vi "ServiceStatusSignals.Compile.vi"(8 "error in (no error)":errorcluster, 10 "Settings":T1[](array[typedef]) {"Signal.Cmd.Refs"."Signal Refs" format="%.0x"; "Signal.Cmd.Info"."Signals"."Byte Order" items=["Little Endian", "Big Endian"]; "Signal.Cmd.Info"."Signals"."Data Type" items=["Signed", "Unsigned", "IEEE Float"]; "Settings.Refs"."Signal Refs" format="%.0x"; "Signal.Resp.Refs"."Signal Refs" format="%.0x"; "Signal.Resp.Info"."Signals"."Byte Order" items=["Little Endian", "Big Endian"]; "Signal.Resp.Info"."Signals"."Data Type" items=["Signed", "Unsigned", "IEEE Float"]; "Trigger.Refs"."Signal Refs" format="%.0x"; "Status.Refs"."Signal Refs" format="%.0x"}) -> (0 "error out":errorcluster, 2 "Refs":T7 {"VS Refs" format="%.0x"}, 3 "Status Lookup":variant)   [LabVIEW 2019, in "Diagnostics Addon System Explorer.lvlib"]
uses:
  Diagnostics Addon System Explorer.lvlib
  <vilib>/NI VeriStand/Custom Device API/Custom Device Item Ref.ctl
  Types/Service.Export.ctl
  Types/Frame.Ref.ctl
  Addon Shared/Types/Type.ctl
  Addon Shared/Types/Frame.Compile.ctl
  Addon Shared/Types/Signal.ctl
  Addon Shared/Types/ServiceChannels.LookupType.ctl
  Addon Shared/SubVIs/Constants.vi
  <vilib>/NI VeriStand/Custom Device API/Custom Device API.lvlib
  Addon Shared/Diagnostics Addon Shared.lvlib
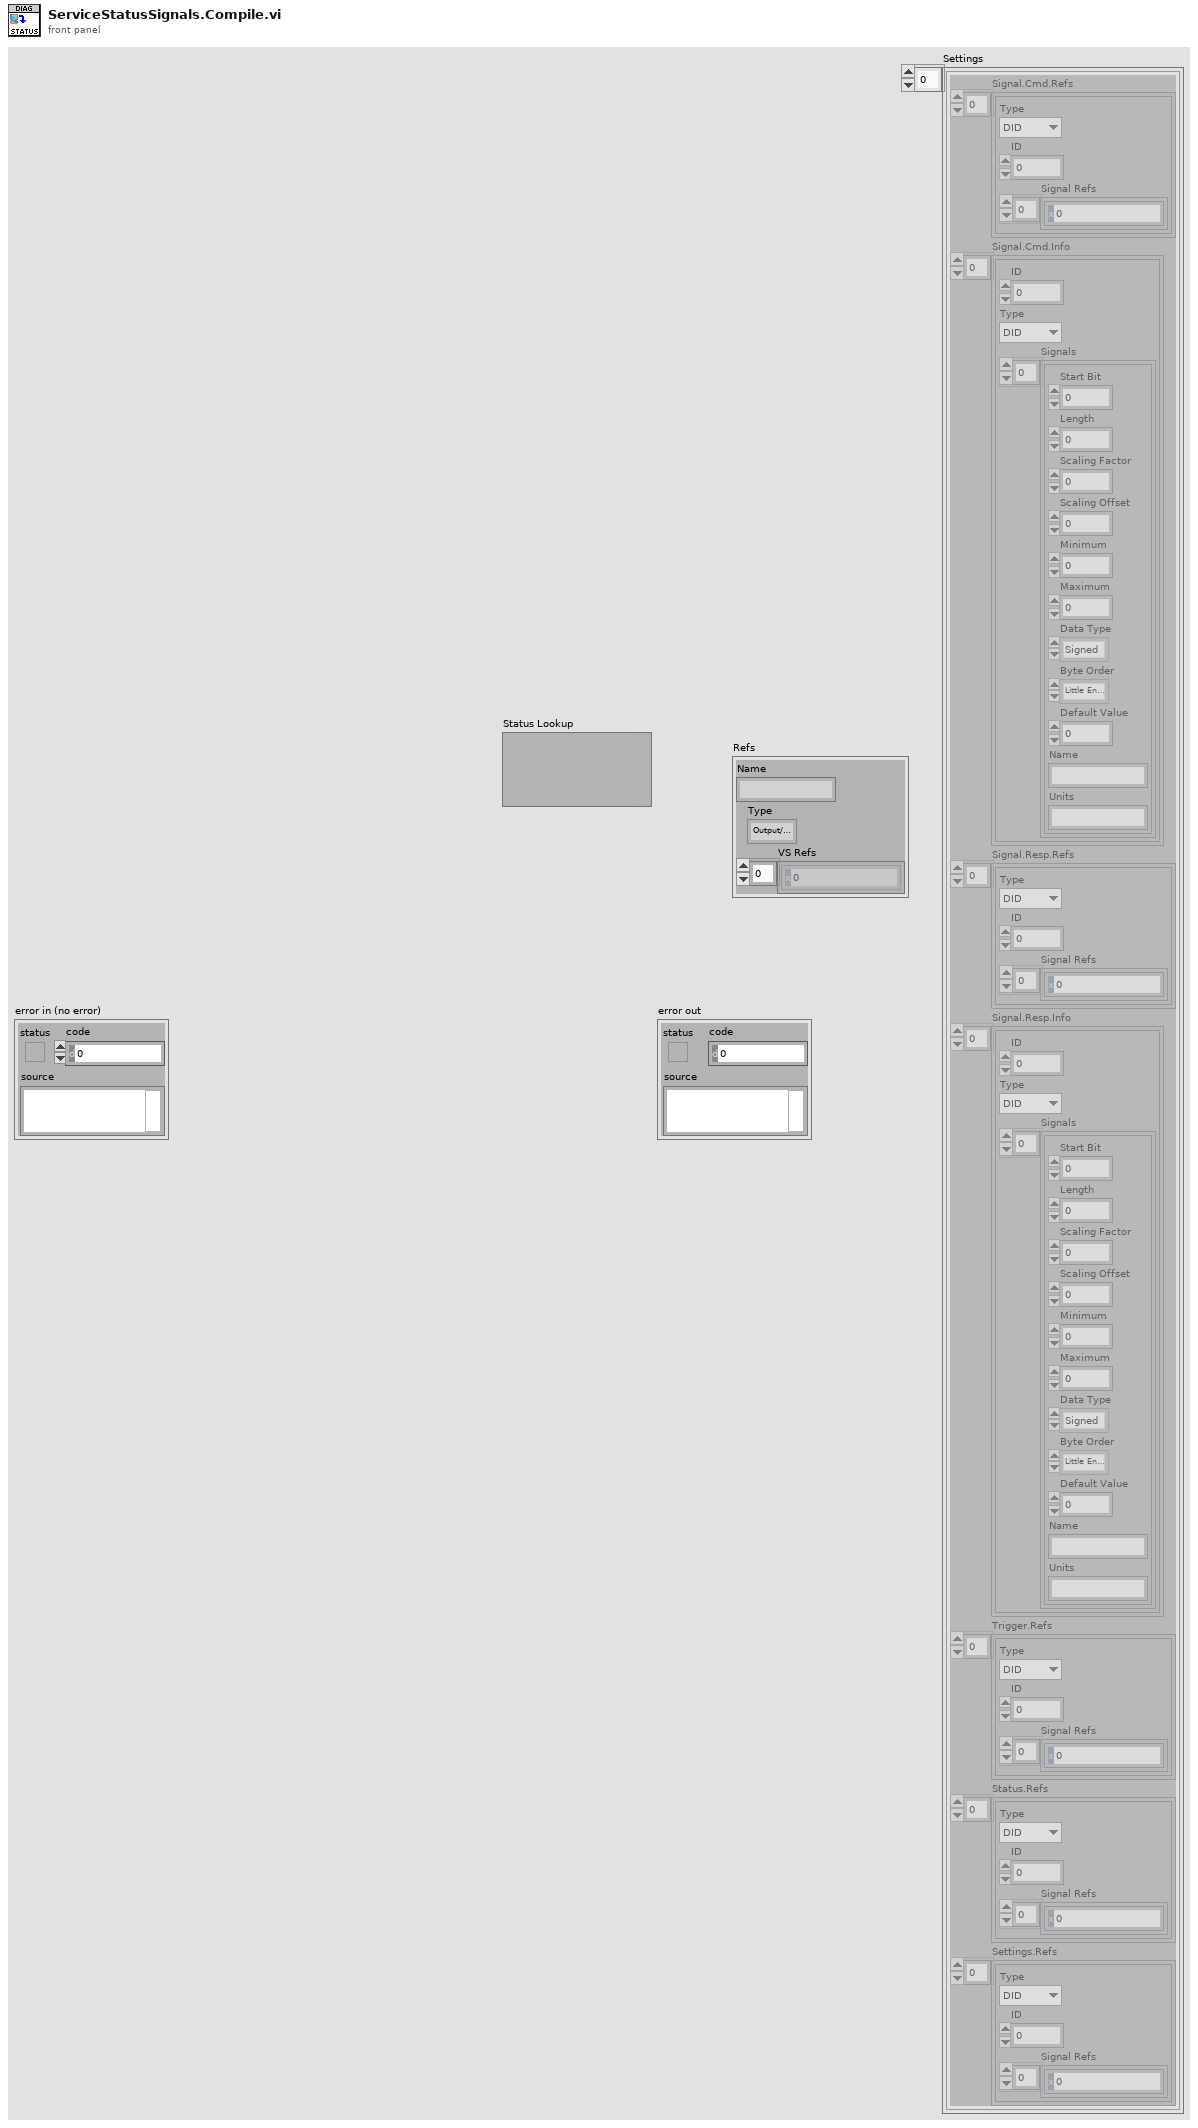
[diagram p1: front panel]
types:
  T1 = typedef "Diagnostics Addon System Explorer.lvlib/Service.Export.ctl" = cluster{"Signal.Cmd.Refs":T2[], "Signal.Cmd.Info":T5[], "Signal.Resp.Refs":T2[], "Signal.Resp.Info":T5[], "Trigger.Refs":T2[], "Status.Refs":T2[], "Settings.Refs":T2[]}
  T2 = typedef "Diagnostics Addon System Explorer.lvlib/Frame.Ref.ctl" = cluster{"Type":T3, "ID":u32, "Signal Refs":T4[]}
  T3 = typedef "Diagnostics Addon Shared.lvlib/Type.ctl" = enum16{"DID", "CDID", "PID", "CPID", "Read Memory", "Write Memory", "IO Control", "Routine Start", "Routine Request", "Routine Stop", "User Defined", "DTC Control", "Clear DTCs", "Read DTCs", "Start DTCs", "DTC Change Count", "Tester Present", "Unlock ECU", "Reset ECU", "Diag Session Control", "Communication Control", "DPID Control", "Poll Control", "Diag CAN Control"}
  T4 = typedef "Custom Device API.lvlib/Custom Device Item Ref.ctl" = u64
  T5 = typedef "Diagnostics Addon Shared.lvlib/Frame.Compile.ctl" = cluster{"ID":u32, "Type":T3, "Signals":T6[]}
  T6 = typedef "Diagnostics Addon Shared.lvlib/Signal.ctl" = cluster{"Start Bit":u32, "Length":u32, "Scaling Factor":dbl, "Scaling Offset":dbl, "Minimum":dbl, "Maximum":dbl, "Data Type":u32, "Byte Order":u32, "Default Value":dbl, "Name":string, "Units":string}
  T7 = cluster{"Name":string, "Type":enum16{"Output/Write", "Input/Read", "Input/ReadWrite"}, "VS Refs":T4[]}
  T8 = enum16{"Output/Write", "Input/Read", "Input/ReadWrite"}
  T9 = typedef "Diagnostics Addon Shared.lvlib/ServiceChannels.LookupType.ctl" = cluster{"Offset":i32}
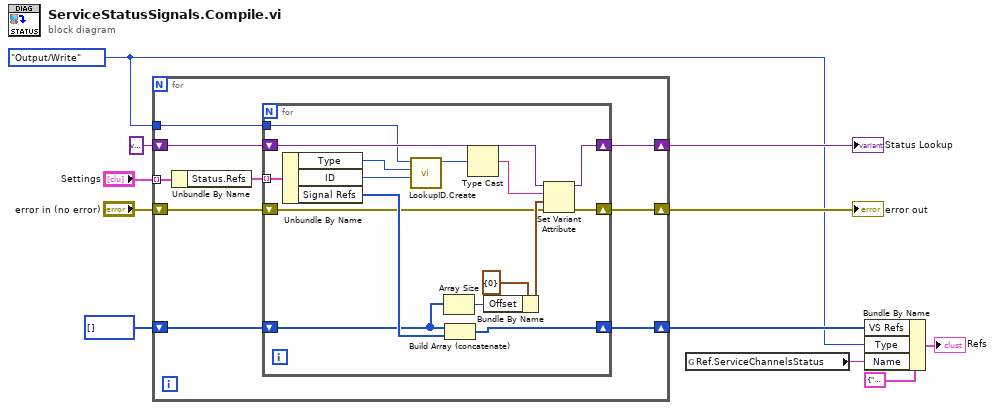
[diagram p0: block diagram]
diagram:
  w1 = T8."Output/Write" ("Type")
  n1 = for {
    shift-right: [w15] -> w4
    shift-left: "error in (no error)" -> [w20]
    shift-right: [w19] -> w10
    shift-left: variant ("Lookup In") -> [w17]
    shift-right: [w16] -> w5
    shift-left: T4[] [] -> [w18]
    tunnel: "Settings" -> [w14] mode=indexing
    tunnel: w1 -> [w12]
    n2 = Unbundle By Name(w14) -> ("Status.Refs"=w13:T2[])
    n3 = for {
      tunnel: w13 -> [w30] mode=indexing
      shift-right: [w31] -> w19
      shift-left: w17 -> [w35]
      shift-right: [w33] -> w15
      shift-left: w20 -> [w26]
      shift-right: [w29] -> w16
      shift-left: w18 -> [w27]
      tunnel: w12 -> [w23]
      n4 = Unbundle By Name(w30) -> ("Type"=w22:T3, "ID"=w24:u32, "Signal Refs"=w28:T4[])
      n5 = call "LookupID.Create.vi"("Serivce ID"=w24, "Service Type"=w22, "Direction"=w23) -> ("Result"=w21:u64)  [unwired: 8 in]
      n6 = Array Size(array=w27) -> (size(s)=w34:i32)
      n7 = Build Array (concatenate)(w27, w28) -> (w29:T4[])
      n8 = Type Cast(x=w21) -> (*(type *) &x=w32:string)  [unwired: 1 in]
      n9 = Bundle By Name(cluster=T9 {"Offset"=0}, "Offset"=w34) -> (w36:T9)
      n10 = Set Variant Attribute(Variant=w35, name=w32, value=w36, error in=w26) -> (Variant out=w31:variant, error out=w33:errorcluster)  [unwired: 1 out]
    }
  }
  "error out" <- w4
  "Status Lookup" <- w10
  n11 = global read "Constants.vi" "Ref.ServiceChannelsStatus"() -> (w7:string)
  n12 = Bundle By Name(cluster=T7 {"Name"="", "Type"=enum."Output/Write", "VS Refs"=[]} ("Group"), "VS Refs"=w5, "Type"=w1, "Name"=w7) -> (→"Refs":T7)
